vi "PanelA.vi"(0 "VI Path":path, 5 "error in (no error)":errorcluster) -> (4 "Controls":T2(array[cluster]), 6 "Indicators":T3[](array[typedef]), 8 "error out":errorcluster)   [LabVIEW 2020]
doc: "This VI displays the controls and indicators of the selected VI in the VI Path."
uses:
  Typedefs/Cluster.ctl
  <vilib>/Utility/Data Type/Type Definitions/Data Type.ctl
  <vilib>/Utility/Data Type/NI_Data Type.lvlib
panel:
  # "Select .vi file in the VI Path then the controls and indicators if the selected \nVI will be displayed here."
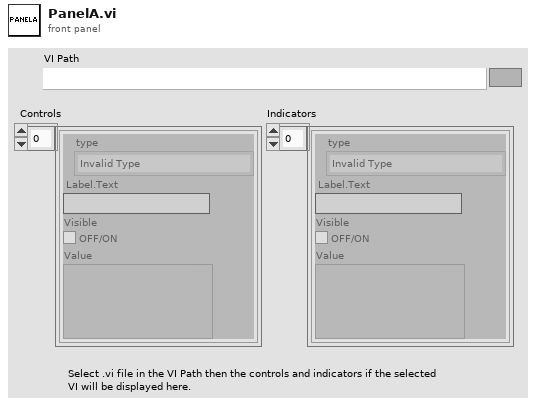
[diagram p1: front panel]
types:
  T1 = typedef "NI_Data Type.lvlib/Data Type.ctl" = enum8{"Invalid Type", "Void", "I8", "I16", "I32", "I64", "U8", "U16", "U32", "U64", "Single Float", "Double Float", "Extended Float", "Single Complex", "Double Complex", "Extended Complex", "Enum U8", "Enum U16", "Enum U32", "Enum U64", "Single Float With Unit", "Double Float With Unit", "Extended Float With Unit", "Single Complex with Unit", "Double Complex with Unit", "Extended Complex with Unit", "Boolean", "String", "Path", "Picture", "Tag", "Array", "Cluster", "Variant", "LV Variant", "Waveform", "Timestamp", "Digital Waveform", "Digital Data", "ExpressData", "Refnum", "External Data", "VI", "Poly VI", "LabVIEW Class Instance", "Fixed Point", "Set Collection", "Map Collection"}
  T2 = cluster{"type":T1, "Label.Text":string, "Visible":bool, "Value":variant}[]
  T3 = typedef "Cluster.ctl" = cluster{"type":T1, "Label.Text":string, "Visible":bool, "Value":variant}
  T4 = cluster{"type":T1, "Label.Text":string, "Visible":bool, "Value":variant}
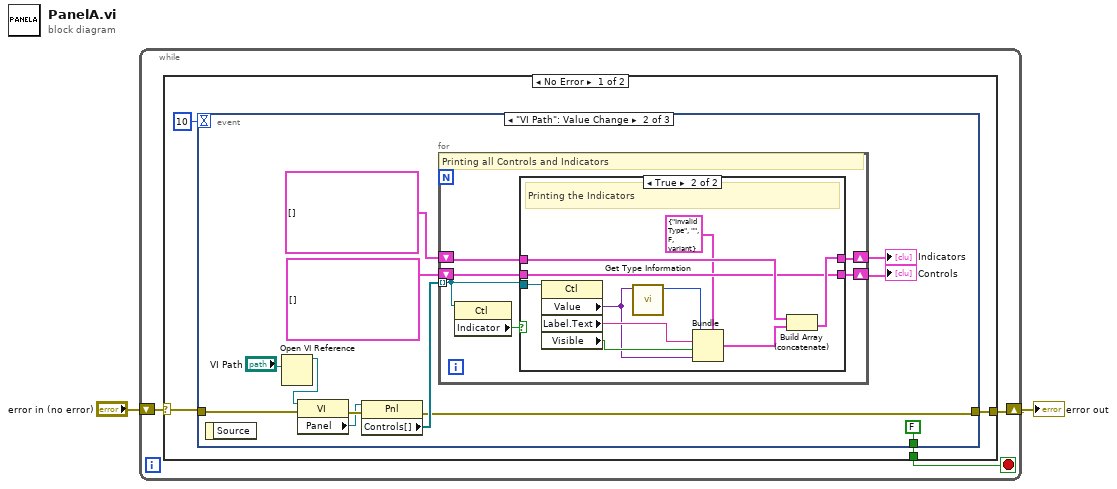
[diagram p0: block diagram]
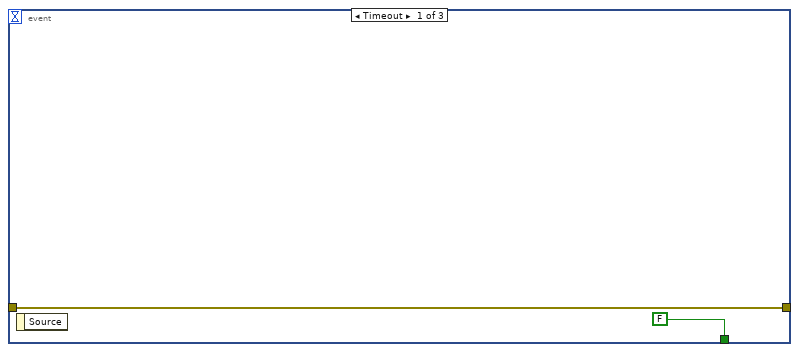
[diagram p2: hidden frame]
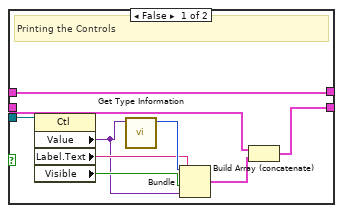
[diagram p3: hidden frame]
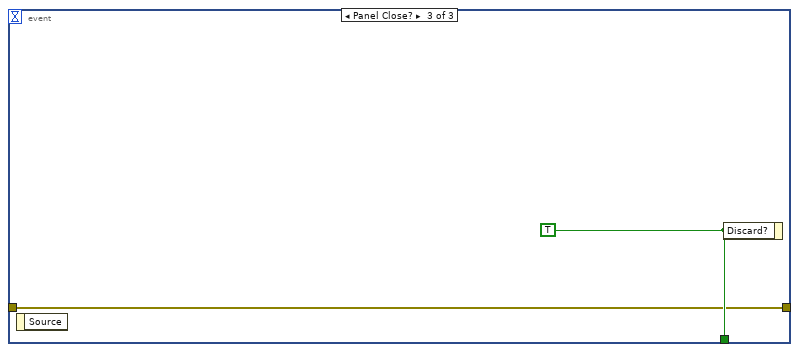
[diagram p4: hidden frame]
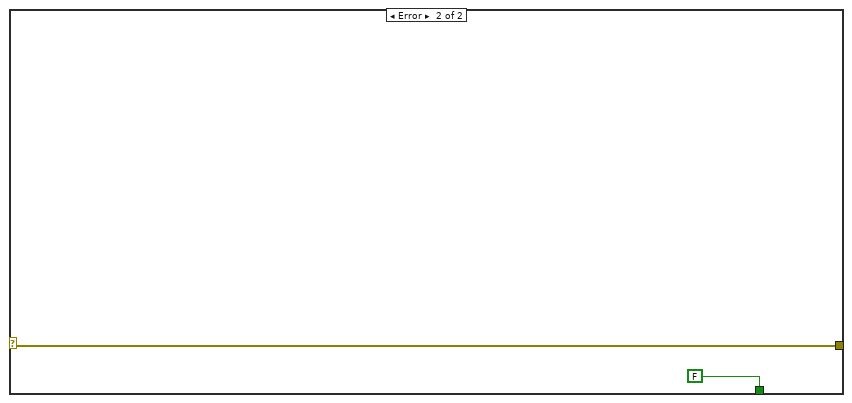
[diagram p5: hidden frame]
diagram:
  n1 = while {
    shift-right: [w5] -> w1
    shift-left: "error in (no error)" -> [w4]
    stop <- w3 stop-if-true
    n2 = case shown="No Error" w4 {
      selector: w4 -> [w8 w52]
      tunnel: [w9 w52] -> w5
      tunnel: [w6 FALSE ("Discard?")] -> w3
      frame No Error {
        n3 = event shown="[1] \"VI Path\": Value Change" {
          selector: _ -> [_ _ _]
          dyn-events: _ -> [_ _ _]
          timeout: 10 -> [_ _ _]
          tunnel: w8 -> [w11 w18 w49]
          tunnel: [w11 w17 w49] -> w9
          tunnel: [FALSE ("Discard?") FALSE ("Discard?") w50] -> w6
          event Timeout {
            n4 = event-data() -> ()  [unwired: 1 in, 1 out]
          }
          event "VI Path": Value Change {
            n5 = event-data() -> ()  [unwired: 1 in, 1 out]
            n6 = Open VI Reference(vi path="VI Path") -> (vi reference=w21:refnum<vi>)  [unwired: 5 in, 1 out]
            n7 = property class="VI"(reference=w21, error in=w18) -> (error out=w23:errorcluster, "Panel"=w19:refnum<vi>)  [unwired: 1 out]
            n8 = property class="Pnl"(reference=w19, error in=w23) -> (error out=w17:errorcluster, "Controls[]"=w20:refnum<vi>[])  [unwired: 1 out]
            n9 = for {
              tunnel: w20 -> [w29] mode=indexing
              shift-right: [w24] -> w15
              shift-left: T3[] [] -> [w27]
              shift-right: [w25] -> w12
              shift-left: T2 [] -> [w26]
              # "Printing all Controls and Indicators"
              n10 = property class="Ctl"(reference=w29) -> ("Indicator"=w28:bool)  [unwired: 1 in, 2 out]
              n11 = case shown="True" w28 {
                tunnel: w29 -> [w37 w47]
                tunnel: w27 -> [w36 w46]
                tunnel: [w36 w45] -> w24
                tunnel: [w38 w44] -> w25
                tunnel: w26 -> [w31 w44]
                frame False {
                  # "Printing the Controls"
                  n12 = property class="Ctl"(reference=w37) -> ("Value"=w32:variant, "Label.Text"=w34:string, "Visible"=w33:bool)  [unwired: 1 in, 2 out]
                  n13 = call <vilib>:"Get Type Information.vi"("variant"=w32) -> ("type"=w35:T1)  [unwired: 6 in, 4 out]
                  n14 = Bundle("type"=w35, "Label.Text"=w34, "Visible"=w33, "Value"=w32) -> (w30:T4)  [unwired: 1 in]
                  n15 = Build Array (concatenate)(w31, w30) -> (w38:T2)
                }
                frame True {
                  # "Printing the Indicators"
                  n16 = property class="Ctl"(reference=w47) -> ("Value"=w41:variant, "Label.Text"=w42:string, "Visible"=w43:bool)  [unwired: 1 in, 2 out]
                  n17 = call <vilib>:"Get Type Information.vi"("variant"=w41) -> ("type"=w48:T1)  [unwired: 6 in, 4 out]
                  n18 = Bundle(cluster=T3 {"type"=enum."Invalid Type", "Label.Text"="", "Visible"=FALSE, "Value"=variant}, "type"=w48, "Label.Text"=w42, "Visible"=w43, "Value"=w41) -> (w40:T3)
                  n19 = Build Array (concatenate)(w46, w40) -> (w45:T3[])
                }
              }
            }
            "Indicators" <- w15
            "Controls" <- w12
          }
          event Panel Close? {
            w50 = TRUE ("Discard?")
            n20 = event-data() -> ()  [unwired: 1 in, 1 out]
            n21 = event-data("Discard?"=w50) -> ()  [unwired: 1 in, 1 out]
          }
        }
      }
      frame Error {
      }
    }
  }
  "error out" <- w1
